vi "36DUT Plot From Spread Sheet.vi"(6 "Plot":T1(ring), 7 "No of Rows":i32=10496, 8 "error in (no error)":errorcluster, 10 "Bank":i32(ring) items=["C1", "C2", "C3", "D_C1", "D_C2", "D_C3"], 11 "file path (dialog if empty)":path) -> (0 "error out":errorcluster, 3 "Delta C_Min Plot":dbl[][](graph) caption="(Y) Multi Plot 2")   [LabVIEW 2012]
uses:
  <vilib>/Utility/file.llb/Read From Spreadsheet File (string).vi
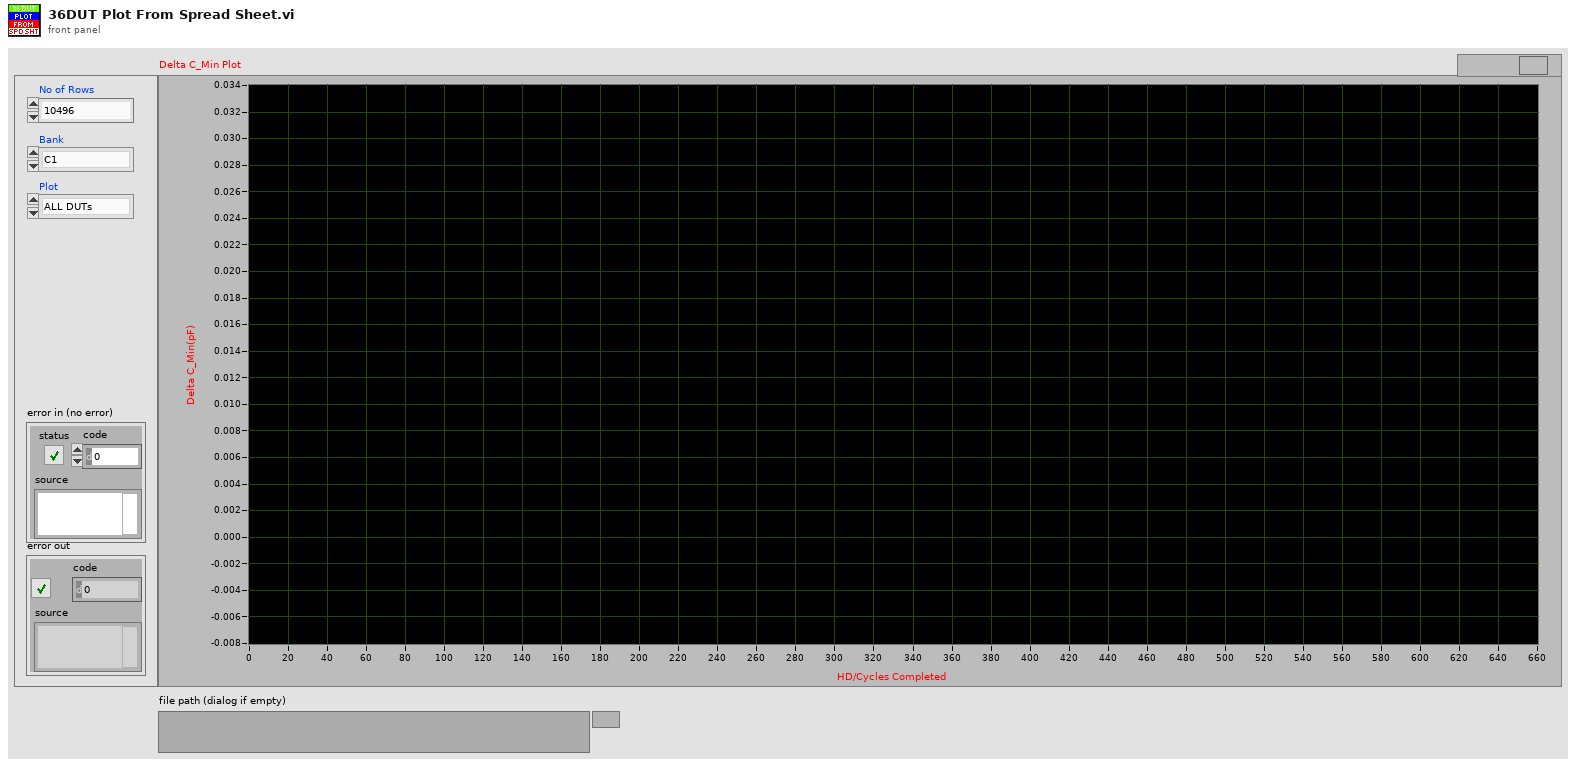
[diagram p1: front panel]
types:
  T1 = enum16{"ALL DUTs", "DUT 01", "DUT 02", "DUT 03", "DUT 04", "DUT 05", "DUT 06", "DUT 07", "DUT 08", "DUT 09", "DUT 10", "DUT 11", "DUT 12", "DUT 13", "DUT 14", "DUT 15", "DUT 16", "DUT 17", "DUT 18", "DUT 19", "DUT 20", "DUT 21", "DUT 22", "DUT 23", "DUT 24", "DUT 25", "DUT 26", "DUT 27", "DUT 28", "DUT 29", "DUT 30", "DUT 31", "DUT 32", "DUT 33", "DUT 34", "DUT 35", "DUT 36"}
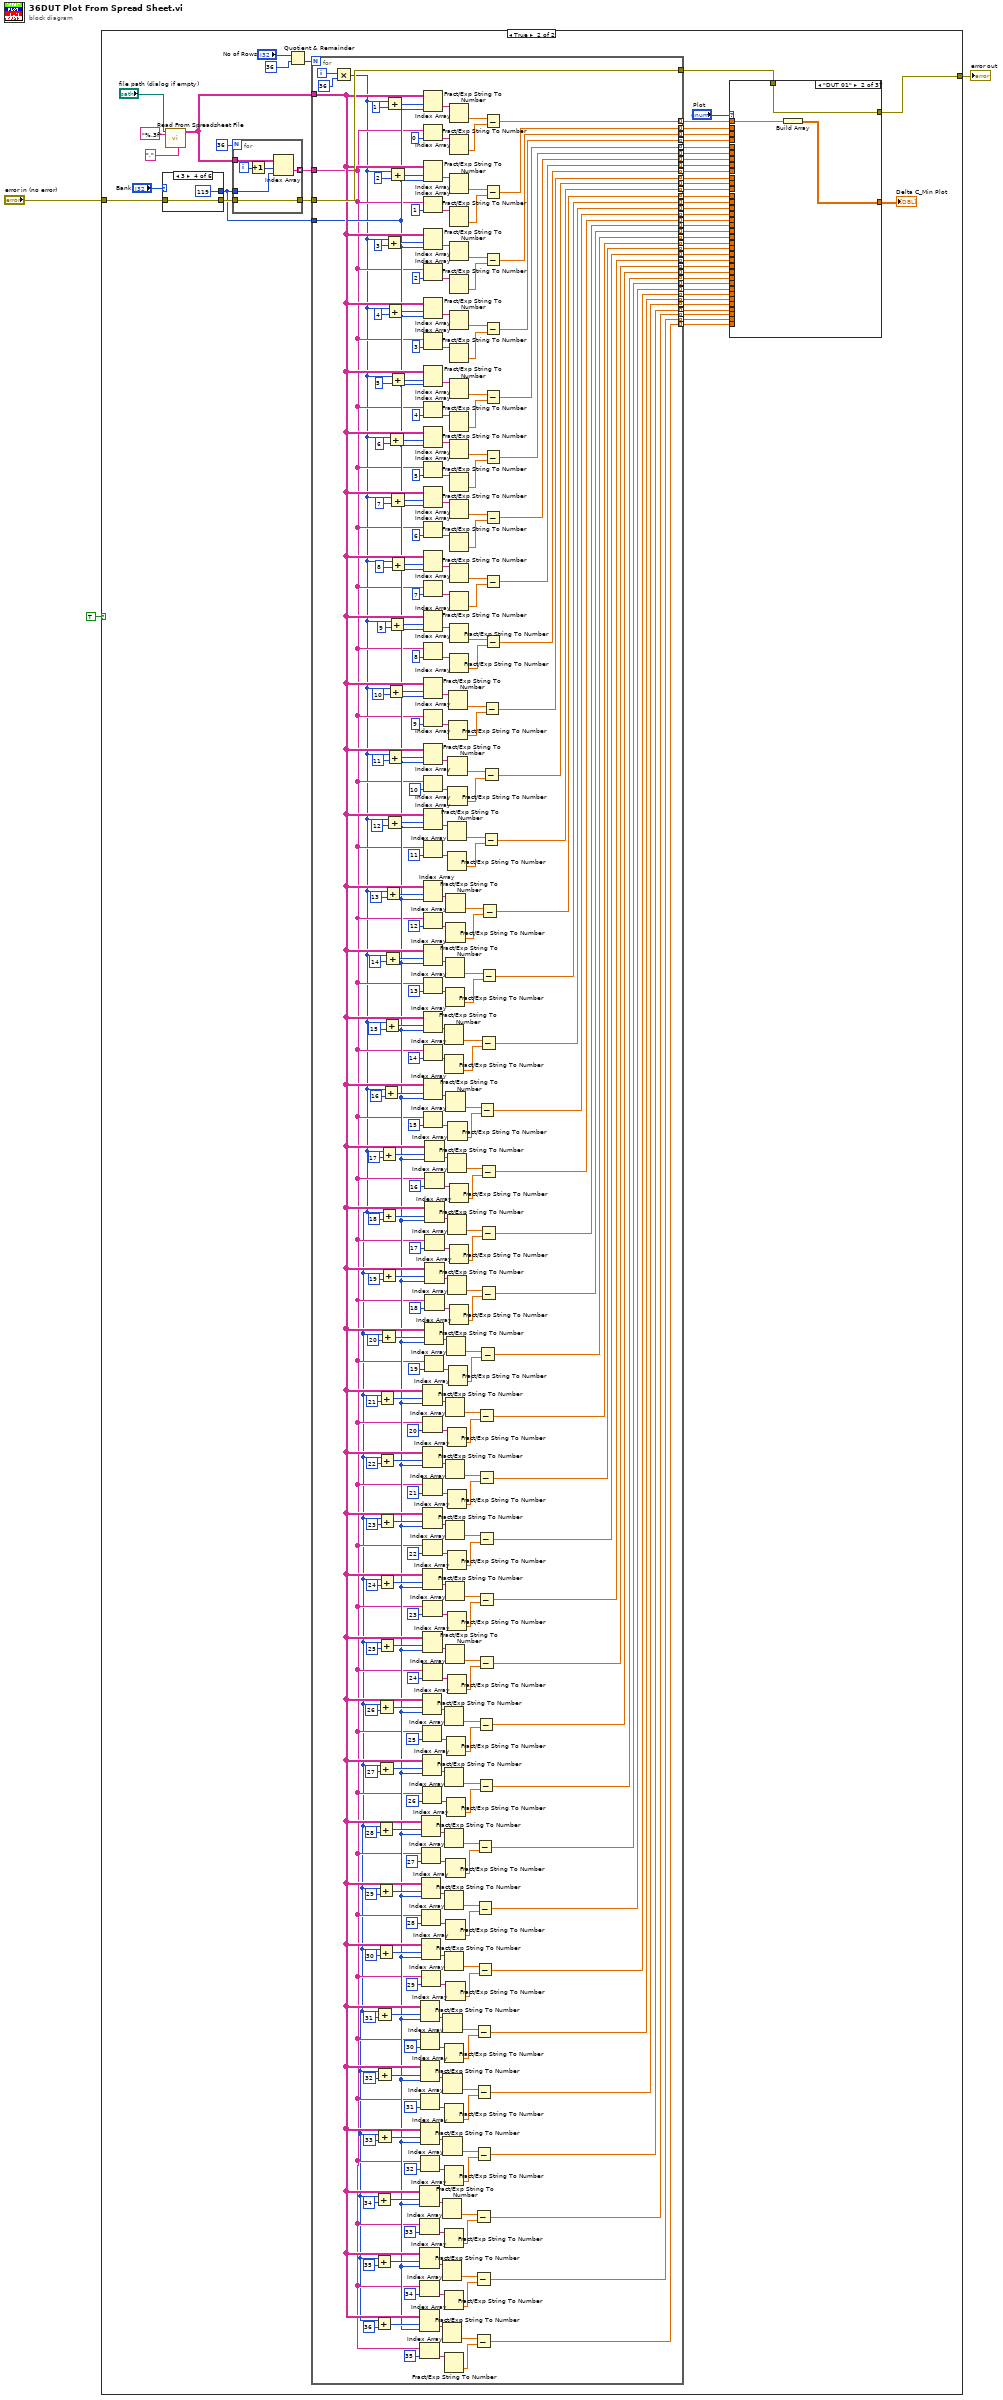
[diagram p0: block diagram]
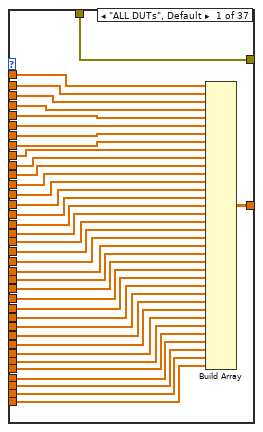
[diagram p3: hidden frame]
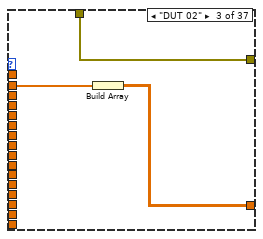
[diagram p4: hidden frame]
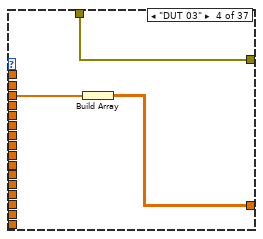
[diagram p5: hidden frame]
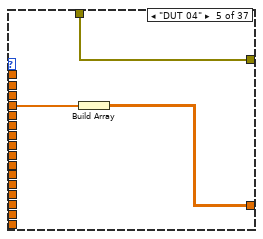
[diagram p6: hidden frame]
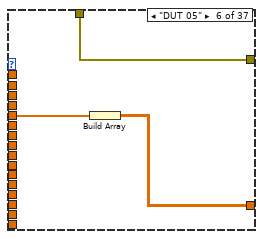
[diagram p7: hidden frame]
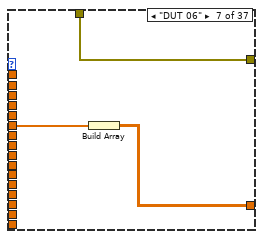
[diagram p8: hidden frame]
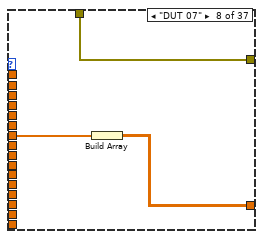
[diagram p9: hidden frame]
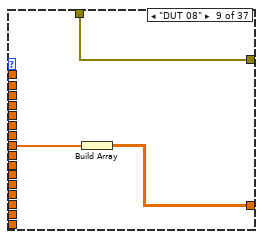
[diagram p10: hidden frame]
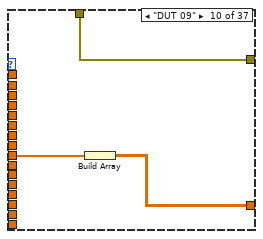
[diagram p11: hidden frame]
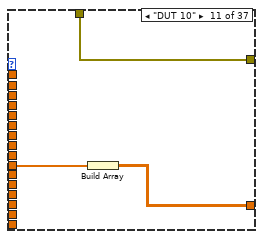
[diagram p12: hidden frame]
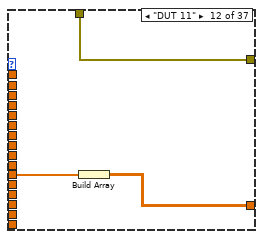
[diagram p13: hidden frame]
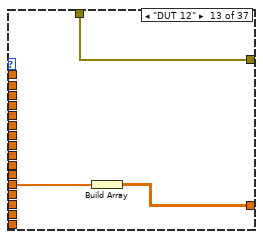
[diagram p14: hidden frame]
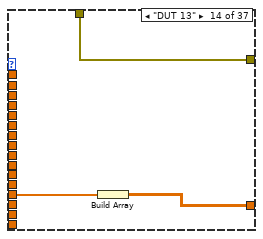
[diagram p15: hidden frame]
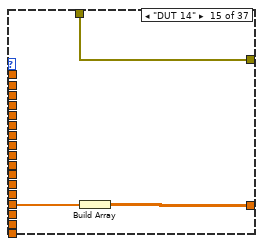
[diagram p16: hidden frame]
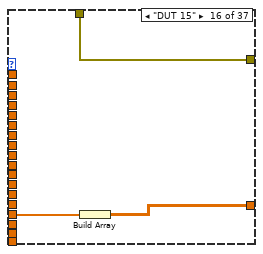
[diagram p17: hidden frame]
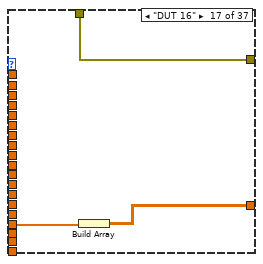
[diagram p18: hidden frame]
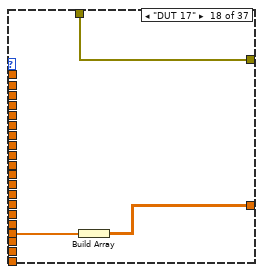
[diagram p19: hidden frame]
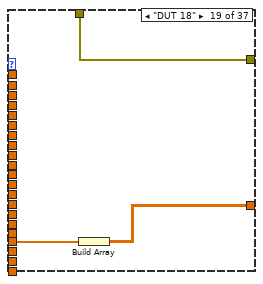
[diagram p20: hidden frame]
diagram:
  n1 = case shown="True" TRUE {
    tunnel: "error in (no error)" -> [w4 w31]
    tunnel: [w4 w25] -> w2
    frame False {
    }
    frame True {
      n2 = case shown="3" "Bank" {
        tunnel: [5 40 75 119 120 121] -> w27
        tunnel: [w205 w207 w209 w212 w214 w216] -> w28
        tunnel: w31 -> [w205 w207 w209 w212 w214 w216]
        frame 0, Default {
        }
        frame 1 {
        }
        frame 2 {
        }
        frame 3 {
        }
        frame 4 {
        }
        frame 5 {
        }
      }
      n3 = call-poly <vilib>:"Read From Spreadsheet File.vi"("delimiter (\\t)"="," ("delimiter (\\t)"), "format (%s)"="%.3f" ("format (%.3f)"), "file path (dialog if empty)"="file path (dialog if empty)") -> ("all rows"=w55:string[][])  [unwired: 4 in, 4 out]
      n4 = for {
        N: 36 -> [_]
        tunnel: w55 -> [w517]
        tunnel: [w516] -> w54 mode=indexing
        tunnel: w27 -> [w512]
        tunnel: [w513] -> w30
        tunnel: w28 -> [w513]
        i -> [w515]
        n5 = Increment(x=w515) -> (x+1=w514:i32)
        n6 = Index Array(array=w517, index (row)=w514, index (col)=w512) -> (element=w516:string)
      }
      n7 = Quotient & Remainder(x="No of Rows", y=36) -> (floor(x/y)=w50:i32)  [unwired: 1 out]
      n8 = for {
        N: w50 -> [_]
        tunnel: w55 -> [w240]
        tunnel: w54 -> [w238]
        tunnel: [w398] -> w48 mode=indexing
        tunnel: [w397] -> w47 mode=indexing
        tunnel: [w396] -> w46 mode=indexing
        tunnel: [w395] -> w45 mode=indexing
        tunnel: [w394] -> w44 mode=indexing
        tunnel: [w393] -> w43 mode=indexing
        tunnel: [w392] -> w42 mode=indexing
        tunnel: [w391] -> w41 mode=indexing
        tunnel: [w390] -> w40 mode=indexing
        tunnel: [w389] -> w39 mode=indexing
        tunnel: [w388] -> w38 mode=indexing
        tunnel: [w387] -> w37 mode=indexing
        tunnel: [w386] -> w36 mode=indexing
        tunnel: [w385] -> w35 mode=indexing
        tunnel: [w384] -> w34 mode=indexing
        tunnel: [w383] -> w33 mode=indexing
        tunnel: w30 -> [w382]
        tunnel: [w382] -> w29
        tunnel: w27 -> [w239]
        tunnel: [w237] -> w24 mode=indexing
        tunnel: [w236] -> w23 mode=indexing
        tunnel: [w235] -> w22 mode=indexing
        tunnel: [w234] -> w21 mode=indexing
        tunnel: [w233] -> w20 mode=indexing
        tunnel: [w232] -> w19 mode=indexing
        tunnel: [w231] -> w18 mode=indexing
        tunnel: [w230] -> w17 mode=indexing
        tunnel: [w229] -> w16 mode=indexing
        tunnel: [w228] -> w15 mode=indexing
        tunnel: [w227] -> w14 mode=indexing
        tunnel: [w226] -> w13 mode=indexing
        tunnel: [w225] -> w12 mode=indexing
        tunnel: [w224] -> w11 mode=indexing
        tunnel: [w223] -> w10 mode=indexing
        tunnel: [w222] -> w9 mode=indexing
        tunnel: [w221] -> w8 mode=indexing
        tunnel: [w220] -> w7 mode=indexing
        tunnel: [w219] -> w6 mode=indexing
        tunnel: [w218] -> w5 mode=indexing
        i -> [w381]
        n9 = Multiply(x=w381, y=36) -> (x*y=w217:i32)
        n10 = Add(x=w217, y=34) -> (x+y=w261:i32)
        n11 = Add(x=w217, y=35) -> (x+y=w248:i32)
        n12 = Add(x=w217, y=36) -> (x+y=w247:i32)
        n13 = Add(x=w217, y=31) -> (x+y=w276:i32)
        n14 = Add(x=w217, y=32) -> (x+y=w275:i32)
        n15 = Add(x=w217, y=33) -> (x+y=w262:i32)
        n16 = Add(x=w217, y=28) -> (x+y=w303:i32)
        n17 = Add(x=w217, y=29) -> (x+y=w290:i32)
        n18 = Add(x=w217, y=30) -> (x+y=w289:i32)
        n19 = Add(x=w217, y=26) -> (x+y=w317:i32)
        n20 = Add(x=w217, y=27) -> (x+y=w304:i32)
        n21 = Add(x=w217, y=21) -> (x+y=w346:i32)
        n22 = Add(x=w217, y=22) -> (x+y=w345:i32)
        n23 = Add(x=w217, y=23) -> (x+y=w332:i32)
        n24 = Add(x=w217, y=24) -> (x+y=w331:i32)
        n25 = Add(x=w217, y=25) -> (x+y=w318:i32)
        n26 = Add(x=w217, y=20) -> (x+y=w359:i32)
        n27 = Add(x=w217, y=17) -> (x+y=w374:i32)
        n28 = Add(x=w217, y=18) -> (x+y=w373:i32)
        n29 = Add(x=w217, y=19) -> (x+y=w360:i32)
        n30 = Add(x=w217, y=16) -> (x+y=w403:i32)
        n31 = Add(x=w217, y=15) -> (x+y=w408:i32)
        n32 = Add(x=w217, y=14) -> (x+y=w417:i32)
        n33 = Add(x=w217, y=13) -> (x+y=w422:i32)
        n34 = Add(x=w217, y=3) -> (x+y=w477:i32)
        n35 = Add(x=w217, y=1) -> (x+y=w499:i32)
        n36 = Add(x=w217, y=12) -> (x+y=w431:i32)
        n37 = Add(x=w217, y=4) -> (x+y=w476:i32)
        n38 = Add(x=w217, y=11) -> (x+y=w436:i32)
        n39 = Add(x=w217, y=10) -> (x+y=w445:i32)
        n40 = Add(x=w217, y=6) -> (x+y=w462:i32)
        n41 = Add(x=w217, y=9) -> (x+y=w492:i32)
        n42 = Add(x=w217, y=2) -> (x+y=w496:i32)
        n43 = Add(x=w217, y=7) -> (x+y=w455:i32)
        n44 = Add(x=w217, y=5) -> (x+y=w469:i32)
        n45 = Add(x=w217, y=8) -> (x+y=w449:i32)
        n46 = Index Array(array=w240, index (row)=w261, index (col)=w239) -> (element=w256:string)
        n47 = Index Array(array=w238, index=33) -> (element=w258:string)
        n48 = Index Array(array=w240, index (row)=w248, index (col)=w239) -> (element=w253:string)
        n49 = Index Array(array=w238, index=34) -> (element=w251:string)
        n50 = Index Array(array=w240, index (row)=w247, index (col)=w239) -> (element=w242:string)
        n51 = Index Array(array=w238, index=35) -> (element=w244:string)
        n52 = Index Array(array=w240, index (row)=w276, index (col)=w239) -> (element=w281:string)
        n53 = Index Array(array=w238, index=30) -> (element=w279:string)
        n54 = Index Array(array=w240, index (row)=w275, index (col)=w239) -> (element=w270:string)
        n55 = Index Array(array=w238, index=31) -> (element=w272:string)
        n56 = Index Array(array=w240, index (row)=w262, index (col)=w239) -> (element=w267:string)
        n57 = Index Array(array=w238, index=32) -> (element=w265:string)
        n58 = Index Array(array=w240, index (row)=w303, index (col)=w239) -> (element=w298:string)
        n59 = Index Array(array=w238, index=27) -> (element=w300:string)
        n60 = Index Array(array=w240, index (row)=w290, index (col)=w239) -> (element=w295:string)
        n61 = Index Array(array=w238, index=28) -> (element=w293:string)
        n62 = Index Array(array=w240, index (row)=w289, index (col)=w239) -> (element=w284:string)
        n63 = Index Array(array=w238, index=29) -> (element=w286:string)
        n64 = Index Array(array=w240, index (row)=w317, index (col)=w239) -> (element=w312:string)
        n65 = Index Array(array=w238, index=25) -> (element=w314:string)
        n66 = Index Array(array=w240, index (row)=w304, index (col)=w239) -> (element=w309:string)
        n67 = Index Array(array=w238, index=26) -> (element=w307:string)
        n68 = Index Array(array=w240, index (row)=w346, index (col)=w239) -> (element=w351:string)
        n69 = Index Array(array=w238, index=20) -> (element=w349:string)
        n70 = Index Array(array=w240, index (row)=w345, index (col)=w239) -> (element=w340:string)
        n71 = Index Array(array=w238, index=21) -> (element=w342:string)
        n72 = Index Array(array=w240, index (row)=w332, index (col)=w239) -> (element=w337:string)
        n73 = Index Array(array=w238, index=22) -> (element=w335:string)
        n74 = Index Array(array=w240, index (row)=w331, index (col)=w239) -> (element=w326:string)
        n75 = Index Array(array=w238, index=23) -> (element=w328:string)
        n76 = Index Array(array=w240, index (row)=w318, index (col)=w239) -> (element=w323:string)
        n77 = Index Array(array=w238, index=24) -> (element=w321:string)
        n78 = Index Array(array=w240, index (row)=w499, index (col)=w239) -> (element=w510:string)
        n79 = Index Array(array=w238, index=0) -> (element=w508:string)
        n80 = Index Array(array=w240, index (row)=w496, index (col)=w239) -> (element=w501:string)
        n81 = Index Array(array=w238, index=1) -> (element=w503:string)
        n82 = Index Array(array=w240, index (row)=w477, index (col)=w239) -> (element=w489:string)
        n83 = Index Array(array=w238, index=2) -> (element=w487:string)
        n84 = Index Array(array=w240, index (row)=w476, index (col)=w239) -> (element=w479:string)
        n85 = Index Array(array=w238, index=3) -> (element=w481:string)
        n86 = Index Array(array=w240, index (row)=w469, index (col)=w239) -> (element=w475:string)
        n87 = Index Array(array=w238, index=4) -> (element=w473:string)
        n88 = Index Array(array=w240, index (row)=w462, index (col)=w239) -> (element=w464:string)
        n89 = Index Array(array=w238, index=5) -> (element=w466:string)
        n90 = Index Array(array=w240, index (row)=w455, index (col)=w239) -> (element=w461:string)
        n91 = Index Array(array=w238, index=6) -> (element=w459:string)
        n92 = Index Array(array=w240, index (row)=w449, index (col)=w239) -> (element=w448:string)
        n93 = Index Array(array=w238, index=7) -> (element=w452:string)
        n94 = Index Array(array=w240, index (row)=w492, index (col)=w239) -> (element=w495:string)
        n95 = Index Array(array=w238, index=8) -> (element=w493:string)
        n96 = Index Array(array=w240, index (row)=w445, index (col)=w239) -> (element=w442:string)
        n97 = Index Array(array=w238, index=9) -> (element=w444:string)
        n98 = Index Array(array=w240, index (row)=w436, index (col)=w239) -> (element=w439:string)
        n99 = Index Array(array=w238, index=10) -> (element=w437:string)
        n100 = Index Array(array=w240, index (row)=w431, index (col)=w239) -> (element=w428:string)
        n101 = Index Array(array=w238, index=11) -> (element=w430:string)
        n102 = Index Array(array=w240, index (row)=w422, index (col)=w239) -> (element=w425:string)
        n103 = Index Array(array=w238, index=12) -> (element=w423:string)
        n104 = Index Array(array=w240, index (row)=w417, index (col)=w239) -> (element=w414:string)
        n105 = Index Array(array=w238, index=13) -> (element=w416:string)
        n106 = Index Array(array=w240, index (row)=w408, index (col)=w239) -> (element=w411:string)
        n107 = Index Array(array=w238, index=14) -> (element=w409:string)
        n108 = Index Array(array=w240, index (row)=w403, index (col)=w239) -> (element=w400:string)
        n109 = Index Array(array=w238, index=15) -> (element=w402:string)
        n110 = Index Array(array=w240, index (row)=w359, index (col)=w239) -> (element=w354:string)
        n111 = Index Array(array=w238, index=19) -> (element=w356:string)
        n112 = Index Array(array=w240, index (row)=w374, index (col)=w239) -> (element=w379:string)
        n113 = Index Array(array=w238, index=16) -> (element=w377:string)
        n114 = Index Array(array=w240, index (row)=w373, index (col)=w239) -> (element=w368:string)
        n115 = Index Array(array=w238, index=17) -> (element=w370:string)
        n116 = Index Array(array=w240, index (row)=w360, index (col)=w239) -> (element=w365:string)
        n117 = Index Array(array=w238, index=18) -> (element=w363:string)
        n118 = Fract/Exp String To Number(string=w256) -> (number=w259:dbl)  [unwired: 3 in, 1 out]
        n119 = Fract/Exp String To Number(string=w253) -> (number=w250:dbl)  [unwired: 3 in, 1 out]
        n120 = Fract/Exp String To Number(string=w242) -> (number=w245:dbl)  [unwired: 3 in, 1 out]
        n121 = Fract/Exp String To Number(string=w281) -> (number=w278:dbl)  [unwired: 3 in, 1 out]
        n122 = Fract/Exp String To Number(string=w270) -> (number=w273:dbl)  [unwired: 3 in, 1 out]
        n123 = Fract/Exp String To Number(string=w267) -> (number=w264:dbl)  [unwired: 3 in, 1 out]
        n124 = Fract/Exp String To Number(string=w298) -> (number=w301:dbl)  [unwired: 3 in, 1 out]
        n125 = Fract/Exp String To Number(string=w295) -> (number=w292:dbl)  [unwired: 3 in, 1 out]
        n126 = Fract/Exp String To Number(string=w284) -> (number=w287:dbl)  [unwired: 3 in, 1 out]
        n127 = Fract/Exp String To Number(string=w258) -> (number=w260:dbl)  [unwired: 3 in, 1 out]
        n128 = Fract/Exp String To Number(string=w251) -> (number=w249:dbl)  [unwired: 3 in, 1 out]
        n129 = Fract/Exp String To Number(string=w244) -> (number=w246:dbl)  [unwired: 3 in, 1 out]
        n130 = Fract/Exp String To Number(string=w411) -> (number=w407:dbl)  [unwired: 3 in, 1 out]
        n131 = Fract/Exp String To Number(string=w409) -> (number=w406:dbl)  [unwired: 3 in, 1 out]
        n132 = Fract/Exp String To Number(string=w312) -> (number=w315:dbl)  [unwired: 3 in, 1 out]
        n133 = Fract/Exp String To Number(string=w309) -> (number=w306:dbl)  [unwired: 3 in, 1 out]
        n134 = Fract/Exp String To Number(string=w279) -> (number=w277:dbl)  [unwired: 3 in, 1 out]
        n135 = Fract/Exp String To Number(string=w272) -> (number=w274:dbl)  [unwired: 3 in, 1 out]
        n136 = Fract/Exp String To Number(string=w265) -> (number=w263:dbl)  [unwired: 3 in, 1 out]
        n137 = Fract/Exp String To Number(string=w414) -> (number=w418:dbl)  [unwired: 3 in, 1 out]
        n138 = Fract/Exp String To Number(string=w416) -> (number=w419:dbl)  [unwired: 3 in, 1 out]
        n139 = Fract/Exp String To Number(string=w351) -> (number=w348:dbl)  [unwired: 3 in, 1 out]
        n140 = Fract/Exp String To Number(string=w340) -> (number=w343:dbl)  [unwired: 3 in, 1 out]
        n141 = Fract/Exp String To Number(string=w337) -> (number=w334:dbl)  [unwired: 3 in, 1 out]
        n142 = Fract/Exp String To Number(string=w326) -> (number=w329:dbl)  [unwired: 3 in, 1 out]
        n143 = Fract/Exp String To Number(string=w323) -> (number=w320:dbl)  [unwired: 3 in, 1 out]
        n144 = Fract/Exp String To Number(string=w425) -> (number=w421:dbl)  [unwired: 3 in, 1 out]
        n145 = Fract/Exp String To Number(string=w423) -> (number=w420:dbl)  [unwired: 3 in, 1 out]
        n146 = Fract/Exp String To Number(string=w400) -> (number=w404:dbl)  [unwired: 3 in, 1 out]
        n147 = Fract/Exp String To Number(string=w300) -> (number=w302:dbl)  [unwired: 3 in, 1 out]
        n148 = Fract/Exp String To Number(string=w293) -> (number=w291:dbl)  [unwired: 3 in, 1 out]
        n149 = Fract/Exp String To Number(string=w286) -> (number=w288:dbl)  [unwired: 3 in, 1 out]
        n150 = Fract/Exp String To Number(string=w354) -> (number=w357:dbl)  [unwired: 3 in, 1 out]
        n151 = Fract/Exp String To Number(string=w314) -> (number=w316:dbl)  [unwired: 3 in, 1 out]
        n152 = Fract/Exp String To Number(string=w307) -> (number=w305:dbl)  [unwired: 3 in, 1 out]
        n153 = Fract/Exp String To Number(string=w428) -> (number=w432:dbl)  [unwired: 3 in, 1 out]
        n154 = Fract/Exp String To Number(string=w430) -> (number=w433:dbl)  [unwired: 3 in, 1 out]
        n155 = Fract/Exp String To Number(string=w379) -> (number=w376:dbl)  [unwired: 3 in, 1 out]
        n156 = Fract/Exp String To Number(string=w368) -> (number=w371:dbl)  [unwired: 3 in, 1 out]
        n157 = Fract/Exp String To Number(string=w365) -> (number=w362:dbl)  [unwired: 3 in, 1 out]
        n158 = Fract/Exp String To Number(string=w349) -> (number=w347:dbl)  [unwired: 3 in, 1 out]
        n159 = Fract/Exp String To Number(string=w342) -> (number=w344:dbl)  [unwired: 3 in, 1 out]
        n160 = Fract/Exp String To Number(string=w335) -> (number=w333:dbl)  [unwired: 3 in, 1 out]
        n161 = Fract/Exp String To Number(string=w328) -> (number=w330:dbl)  [unwired: 3 in, 1 out]
        n162 = Fract/Exp String To Number(string=w321) -> (number=w319:dbl)  [unwired: 3 in, 1 out]
        n163 = Fract/Exp String To Number(string=w439) -> (number=w435:dbl)  [unwired: 3 in, 1 out]
        n164 = Fract/Exp String To Number(string=w437) -> (number=w434:dbl)  [unwired: 3 in, 1 out]
        n165 = Fract/Exp String To Number(string=w402) -> (number=w405:dbl)  [unwired: 3 in, 1 out]
        n166 = Fract/Exp String To Number(string=w442) -> (number=w446:dbl)  [unwired: 3 in, 1 out]
        n167 = Fract/Exp String To Number(string=w444) -> (number=w447:dbl)  [unwired: 3 in, 1 out]
        n168 = Fract/Exp String To Number(string=w356) -> (number=w358:dbl)  [unwired: 3 in, 1 out]
        n169 = Fract/Exp String To Number(string=w377) -> (number=w375:dbl)  [unwired: 3 in, 1 out]
        n170 = Fract/Exp String To Number(string=w370) -> (number=w372:dbl)  [unwired: 3 in, 1 out]
        n171 = Fract/Exp String To Number(string=w363) -> (number=w361:dbl)  [unwired: 3 in, 1 out]
        n172 = Fract/Exp String To Number(string=w510) -> (number=w507:dbl)  [unwired: 3 in, 1 out]
        n173 = Fract/Exp String To Number(string=w508) -> (number=w506:dbl)  [unwired: 3 in, 1 out]
        n174 = Fract/Exp String To Number(string=w501) -> (number=w504:dbl)  [unwired: 3 in, 1 out]
        n175 = Fract/Exp String To Number(string=w503) -> (number=w505:dbl)  [unwired: 3 in, 1 out]
        n176 = Fract/Exp String To Number(string=w489) -> (number=w486:dbl)  [unwired: 3 in, 1 out]
        n177 = Fract/Exp String To Number(string=w487) -> (number=w485:dbl)  [unwired: 3 in, 1 out]
        n178 = Fract/Exp String To Number(string=w479) -> (number=w482:dbl)  [unwired: 3 in, 1 out]
        n179 = Fract/Exp String To Number(string=w481) -> (number=w483:dbl)  [unwired: 3 in, 1 out]
        n180 = Fract/Exp String To Number(string=w475) -> (number=w472:dbl)  [unwired: 3 in, 1 out]
        n181 = Fract/Exp String To Number(string=w473) -> (number=w471:dbl)  [unwired: 3 in, 1 out]
        n182 = Fract/Exp String To Number(string=w464) -> (number=w467:dbl)  [unwired: 3 in, 1 out]
        n183 = Fract/Exp String To Number(string=w466) -> (number=w468:dbl)  [unwired: 3 in, 1 out]
        n184 = Fract/Exp String To Number(string=w461) -> (number=w458:dbl)  [unwired: 3 in, 1 out]
        n185 = Fract/Exp String To Number(string=w459) -> (number=w457:dbl)  [unwired: 3 in, 1 out]
        n186 = Fract/Exp String To Number(string=w448) -> (number=w453:dbl)  [unwired: 3 in, 1 out]
        n187 = Fract/Exp String To Number(string=w452) -> (number=w454:dbl)  [unwired: 3 in, 1 out]
        n188 = Fract/Exp String To Number(string=w495) -> (number=w491:dbl)  [unwired: 3 in, 1 out]
        n189 = Fract/Exp String To Number(string=w493) -> (number=w490:dbl)  [unwired: 3 in, 1 out]
        n190 = Subtract(x=w259, y=w260) -> (x-y=w220:dbl)
        n191 = Subtract(x=w250, y=w249) -> (x-y=w219:dbl)
        n192 = Subtract(x=w245, y=w246) -> (x-y=w218:dbl)
        n193 = Subtract(x=w278, y=w277) -> (x-y=w223:dbl)
        n194 = Subtract(x=w273, y=w274) -> (x-y=w222:dbl)
        n195 = Subtract(x=w264, y=w263) -> (x-y=w221:dbl)
        n196 = Subtract(x=w301, y=w302) -> (x-y=w226:dbl)
        n197 = Subtract(x=w292, y=w291) -> (x-y=w225:dbl)
        n198 = Subtract(x=w287, y=w288) -> (x-y=w224:dbl)
        n199 = Subtract(x=w315, y=w316) -> (x-y=w228:dbl)
        n200 = Subtract(x=w306, y=w305) -> (x-y=w227:dbl)
        n201 = Subtract(x=w348, y=w347) -> (x-y=w233:dbl)
        n202 = Subtract(x=w343, y=w344) -> (x-y=w232:dbl)
        n203 = Subtract(x=w334, y=w333) -> (x-y=w231:dbl)
        n204 = Subtract(x=w329, y=w330) -> (x-y=w230:dbl)
        n205 = Subtract(x=w320, y=w319) -> (x-y=w229:dbl)
        n206 = Subtract(x=w404, y=w405) -> (x-y=w383:dbl)
        n207 = Subtract(x=w357, y=w358) -> (x-y=w234:dbl)
        n208 = Subtract(x=w407, y=w406) -> (x-y=w384:dbl)
        n209 = Subtract(x=w376, y=w375) -> (x-y=w237:dbl)
        n210 = Subtract(x=w371, y=w372) -> (x-y=w236:dbl)
        n211 = Subtract(x=w362, y=w361) -> (x-y=w235:dbl)
        n212 = Subtract(x=w418, y=w419) -> (x-y=w385:dbl)
        n213 = Subtract(x=w421, y=w420) -> (x-y=w386:dbl)
        n214 = Subtract(x=w432, y=w433) -> (x-y=w387:dbl)
        n215 = Subtract(x=w435, y=w434) -> (x-y=w388:dbl)
        n216 = Subtract(x=w446, y=w447) -> (x-y=w389:dbl)
        n217 = Subtract(x=w507, y=w506) -> (x-y=w398:dbl)
        n218 = Subtract(x=w504, y=w505) -> (x-y=w397:dbl)
        n219 = Subtract(x=w486, y=w485) -> (x-y=w396:dbl)
        n220 = Subtract(x=w482, y=w483) -> (x-y=w395:dbl)
        n221 = Subtract(x=w472, y=w471) -> (x-y=w394:dbl)
        n222 = Subtract(x=w467, y=w468) -> (x-y=w393:dbl)
        n223 = Subtract(x=w458, y=w457) -> (x-y=w392:dbl)
        n224 = Subtract(x=w453, y=w454) -> (x-y=w391:dbl)
        n225 = Subtract(x=w491, y=w490) -> (x-y=w390:dbl)
      }
      n226 = case shown="\"DUT 01\"" "Plot" {
        tunnel: w48 -> [w96 w99 _ _ _ _ _ _ _ _ _ _ _ _ _ _ _ _ _ _ _ _ _ _ _ _ _ _ _ _ _ _ _ _ _ _ _]
        tunnel: w47 -> [w95 _ w101 _ _ _ _ _ _ _ _ _ _ _ _ _ _ _ _ _ _ _ _ _ _ _ _ _ _ _ _ _ _ _ _ _ _]
        tunnel: w46 -> [w94 _ _ w105 _ _ _ _ _ _ _ _ _ _ _ _ _ _ _ _ _ _ _ _ _ _ _ _ _ _ _ _ _ _ _ _ _]
        tunnel: w45 -> [w93 _ _ _ w107 _ _ _ _ _ _ _ _ _ _ _ _ _ _ _ _ _ _ _ _ _ _ _ _ _ _ _ _ _ _ _ _]
        tunnel: w44 -> [w92 _ _ _ _ w111 _ _ _ _ _ _ _ _ _ _ _ _ _ _ _ _ _ _ _ _ _ _ _ _ _ _ _ _ _ _ _]
        tunnel: w43 -> [w91 _ _ _ _ _ w113 _ _ _ _ _ _ _ _ _ _ _ _ _ _ _ _ _ _ _ _ _ _ _ _ _ _ _ _ _ _]
        tunnel: w42 -> [w90 _ _ _ _ _ _ w116 _ _ _ _ _ _ _ _ _ _ _ _ _ _ _ _ _ _ _ _ _ _ _ _ _ _ _ _ _]
        tunnel: w41 -> [w89 _ _ _ _ _ _ _ w120 _ _ _ _ _ _ _ _ _ _ _ _ _ _ _ _ _ _ _ _ _ _ _ _ _ _ _ _]
        tunnel: w40 -> [w88 _ _ _ _ _ _ _ _ w123 _ _ _ _ _ _ _ _ _ _ _ _ _ _ _ _ _ _ _ _ _ _ _ _ _ _ _]
        tunnel: w39 -> [w87 _ _ _ _ _ _ _ _ _ w126 _ _ _ _ _ _ _ _ _ _ _ _ _ _ _ _ _ _ _ _ _ _ _ _ _ _]
        tunnel: w38 -> [w86 _ _ _ _ _ _ _ _ _ _ w129 _ _ _ _ _ _ _ _ _ _ _ _ _ _ _ _ _ _ _ _ _ _ _ _ _]
        tunnel: w37 -> [w85 _ _ _ _ _ _ _ _ _ _ _ w132 _ _ _ _ _ _ _ _ _ _ _ _ _ _ _ _ _ _ _ _ _ _ _ _]
        tunnel: w36 -> [w84 _ _ _ _ _ _ _ _ _ _ _ _ w135 _ _ _ _ _ _ _ _ _ _ _ _ _ _ _ _ _ _ _ _ _ _ _]
        tunnel: w35 -> [w83 _ _ _ _ _ _ _ _ _ _ _ _ _ w138 _ _ _ _ _ _ _ _ _ _ _ _ _ _ _ _ _ _ _ _ _ _]
        tunnel: w34 -> [w82 _ _ _ _ _ _ _ _ _ _ _ _ _ _ w141 _ _ _ _ _ _ _ _ _ _ _ _ _ _ _ _ _ _ _ _ _]
        tunnel: w33 -> [w81 _ _ _ _ _ _ _ _ _ _ _ _ _ _ _ w143 _ _ _ _ _ _ _ _ _ _ _ _ _ _ _ _ _ _ _ _]
        tunnel: [w80 w98 w102 w104 w108 w110 w114 w117 w119 w122 w125 w128 w131 w134 w137 w140 w144 w147 w150 w153 w156 w159 w162 w165 w168 w171 w174 w177 w180 w183 w186 w189 w192 w195 w198 w201 w204] -> w32
        tunnel: w29 -> [w79 w97 w100 w103 w106 w109 w112 w115 w118 w121 w124 w127 w130 w133 w136 w139 w142 w146 w149 w152 w155 w158 w161 w164 w167 w170 w173 w176 w179 w182 w185 w188 w191 w194 w197 w200 w203]
        tunnel: [w79 w97 w100 w103 w106 w109 w112 w115 w118 w121 w124 w127 w130 w133 w136 w139 w142 w146 w149 w152 w155 w158 w161 w164 w167 w170 w173 w176 w179 w182 w185 w188 w191 w194 w197 w200 w203] -> w25
        tunnel: w24 -> [w78 _ _ _ _ _ _ _ _ _ _ _ _ _ _ _ _ w145 _ _ _ _ _ _ _ _ _ _ _ _ _ _ _ _ _ _ _]
        tunnel: w23 -> [w77 _ _ _ _ _ _ _ _ _ _ _ _ _ _ _ _ _ w148 _ _ _ _ _ _ _ _ _ _ _ _ _ _ _ _ _ _]
        tunnel: w22 -> [w76 _ _ _ _ _ _ _ _ _ _ _ _ _ _ _ _ _ _ w151 _ _ _ _ _ _ _ _ _ _ _ _ _ _ _ _ _]
        tunnel: w21 -> [w75 _ _ _ _ _ _ _ _ _ _ _ _ _ _ _ _ _ _ _ w154 _ _ _ _ _ _ _ _ _ _ _ _ _ _ _ _]
        tunnel: w20 -> [w74 _ _ _ _ _ _ _ _ _ _ _ _ _ _ _ _ _ _ _ _ w157 _ _ _ _ _ _ _ _ _ _ _ _ _ _ _]
        tunnel: w19 -> [w73 _ _ _ _ _ _ _ _ _ _ _ _ _ _ _ _ _ _ _ _ _ w160 _ _ _ _ _ _ _ _ _ _ _ _ _ _]
        tunnel: w18 -> [w72 _ _ _ _ _ _ _ _ _ _ _ _ _ _ _ _ _ _ _ _ _ _ w163 _ _ _ _ _ _ _ _ _ _ _ _ _]
        tunnel: w17 -> [w71 _ _ _ _ _ _ _ _ _ _ _ _ _ _ _ _ _ _ _ _ _ _ _ w166 _ _ _ _ _ _ _ _ _ _ _ _]
        tunnel: w16 -> [w70 _ _ _ _ _ _ _ _ _ _ _ _ _ _ _ _ _ _ _ _ _ _ _ _ w169 _ _ _ _ _ _ _ _ _ _ _]
        tunnel: w15 -> [w69 _ _ _ _ _ _ _ _ _ _ _ _ _ _ _ _ _ _ _ _ _ _ _ _ _ w172 _ _ _ _ _ _ _ _ _ _]
        tunnel: w14 -> [w68 _ _ _ _ _ _ _ _ _ _ _ _ _ _ _ _ _ _ _ _ _ _ _ _ _ _ w175 _ _ _ _ _ _ _ _ _]
        tunnel: w13 -> [w67 _ _ _ _ _ _ _ _ _ _ _ _ _ _ _ _ _ _ _ _ _ _ _ _ _ _ _ w178 _ _ _ _ _ _ _ _]
        tunnel: w12 -> [w66 _ _ _ _ _ _ _ _ _ _ _ _ _ _ _ _ _ _ _ _ _ _ _ _ _ _ _ _ w181 _ _ _ _ _ _ _]
        tunnel: w11 -> [w65 _ _ _ _ _ _ _ _ _ _ _ _ _ _ _ _ _ _ _ _ _ _ _ _ _ _ _ _ _ w184 _ _ _ _ _ _]
        tunnel: w10 -> [w64 _ _ _ _ _ _ _ _ _ _ _ _ _ _ _ _ _ _ _ _ _ _ _ _ _ _ _ _ _ _ w187 _ _ _ _ _]
        tunnel: w9 -> [w63 _ _ _ _ _ _ _ _ _ _ _ _ _ _ _ _ _ _ _ _ _ _ _ _ _ _ _ _ _ _ _ w190 _ _ _ _]
        tunnel: w8 -> [w62 _ _ _ _ _ _ _ _ _ _ _ _ _ _ _ _ _ _ _ _ _ _ _ _ _ _ _ _ _ _ _ _ w193 _ _ _]
        tunnel: w7 -> [w61 _ _ _ _ _ _ _ _ _ _ _ _ _ _ _ _ _ _ _ _ _ _ _ _ _ _ _ _ _ _ _ _ _ w196 _ _]
        tunnel: w6 -> [w60 _ _ _ _ _ _ _ _ _ _ _ _ _ _ _ _ _ _ _ _ _ _ _ _ _ _ _ _ _ _ _ _ _ _ w199 _]
        tunnel: w5 -> [w59 _ _ _ _ _ _ _ _ _ _ _ _ _ _ _ _ _ _ _ _ _ _ _ _ _ _ _ _ _ _ _ _ _ _ _ w202]
        frame "ALL DUTs", Default {
          n227 = Build Array(w96, w95, w94, w93, w92, w91, w90, w89, w88, w87, w86, w85, w84, w83, w82, w81, w78, w77, w76, w75, w74, w73, w72, w71, w70, w69, w68, w67, w66, w65, w64, w63, w62, w61, w60, w59) -> (w80:dbl[][])
        }
        frame "DUT 01" {
          n228 = Build Array(w99) -> (w98:dbl[][])
        }
        frame "DUT 02" {
          n229 = Build Array(w101) -> (w102:dbl[][])
        }
        frame "DUT 03" {
          n230 = Build Array(w105) -> (w104:dbl[][])
        }
        frame "DUT 04" {
          n231 = Build Array(w107) -> (w108:dbl[][])
        }
        frame "DUT 05" {
          n232 = Build Array(w111) -> (w110:dbl[][])
        }
        frame "DUT 06" {
          n233 = Build Array(w113) -> (w114:dbl[][])
        }
        frame "DUT 07" {
          n234 = Build Array(w116) -> (w117:dbl[][])
        }
        frame "DUT 08" {
          n235 = Build Array(w120) -> (w119:dbl[][])
        }
        frame "DUT 09" {
          n236 = Build Array(w123) -> (w122:dbl[][])
        }
        frame "DUT 10" {
          n237 = Build Array(w126) -> (w125:dbl[][])
        }
        frame "DUT 11" {
          n238 = Build Array(w129) -> (w128:dbl[][])
        }
        frame "DUT 12" {
          n239 = Build Array(w132) -> (w131:dbl[][])
        }
        frame "DUT 13" {
          n240 = Build Array(w135) -> (w134:dbl[][])
        }
        frame "DUT 14" {
          n241 = Build Array(w138) -> (w137:dbl[][])
        }
        frame "DUT 15" {
          n242 = Build Array(w141) -> (w140:dbl[][])
        }
        frame "DUT 16" {
          n243 = Build Array(w143) -> (w144:dbl[][])
        }
        frame "DUT 17" {
          n244 = Build Array(w145) -> (w147:dbl[][])
        }
        frame "DUT 18" {
          n245 = Build Array(w148) -> (w150:dbl[][])
        }
        frame "DUT 19" {
          n246 = Build Array(w151) -> (w153:dbl[][])
        }
        frame "DUT 20" {
          n247 = Build Array(w154) -> (w156:dbl[][])
        }
        frame "DUT 21" {
          n248 = Build Array(w157) -> (w159:dbl[][])
        }
        frame "DUT 22" {
          n249 = Build Array(w160) -> (w162:dbl[][])
        }
        frame "DUT 23" {
          n250 = Build Array(w163) -> (w165:dbl[][])
        }
        frame "DUT 24" {
          n251 = Build Array(w166) -> (w168:dbl[][])
        }
        frame "DUT 25" {
          n252 = Build Array(w169) -> (w171:dbl[][])
        }
        frame "DUT 26" {
          n253 = Build Array(w172) -> (w174:dbl[][])
        }
        frame "DUT 27" {
          n254 = Build Array(w175) -> (w177:dbl[][])
        }
        frame "DUT 28" {
          n255 = Build Array(w178) -> (w180:dbl[][])
        }
        frame "DUT 29" {
          n256 = Build Array(w181) -> (w183:dbl[][])
        }
        frame "DUT 30" {
          n257 = Build Array(w184) -> (w186:dbl[][])
        }
        frame "DUT 31" {
          n258 = Build Array(w187) -> (w189:dbl[][])
        }
        frame "DUT 32" {
          n259 = Build Array(w190) -> (w192:dbl[][])
        }
        frame "DUT 33" {
          n260 = Build Array(w193) -> (w195:dbl[][])
        }
        frame "DUT 34" {
          n261 = Build Array(w196) -> (w198:dbl[][])
        }
        frame "DUT 35" {
          n262 = Build Array(w199) -> (w201:dbl[][])
        }
        frame "DUT 36" {
          n263 = Build Array(w202) -> (w204:dbl[][])
        }
      }
      "Delta C_Min Plot" <- w32
    }
  }
  "error out" <- w2
